vi "SetScale.vi"(8 "error in (no error)":errorcluster, 9 "Gauss":T1(ring), 10 "Arduino Resource In":T2={"VISA resource"="", "Board Type"=enum."Uno", "Connection Type"=enum."USB / Serial", "Bytes Per Packet (15)"=15}, 11 "HMC5883L in":refnum<class "HMC5883L.lvclass">) -> (0 "error out":errorcluster, 2 "Arduino Resource Out":T2={"VISA resource"="", "Board Type"=enum."Uno", "Connection Type"=enum."USB / Serial", "Bytes Per Packet (15)"=15}, 3 "HMC5883L out":refnum<class "HMC5883L.lvclass">)   [LabVIEW 2012, in "HMC5883L.lvclass"]
uses:
  HMC5883L.lvclass
  <vilib>/LabVIEW Interface for Arduino/LabVIEW Interface for Arduino.lvlib
  <vilib>/LabVIEW Interface for Arduino/Type Defs/Board Type.ctl
  <vilib>/LabVIEW Interface for Arduino/Type Defs/Arduino Resource.ctl
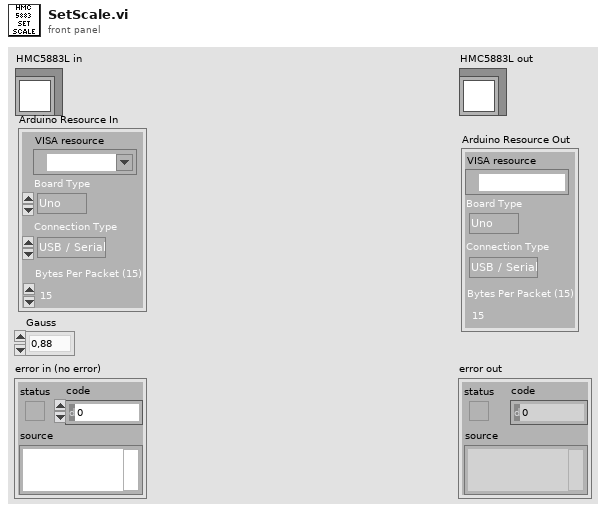
[diagram p1: front panel]
types:
  T1 = enum8{"0,88", "1,30", "1,90", "2,50", "4,00", "4,70", "5,60", "8,10"}
  T2 = typedef "LabVIEW Interface for Arduino.lvlib/Arduino Resource.ctl" = cluster{"VISA resource":refnum<visa-resource-name>, "Board Type":T3, "Connection Type":enum8{"USB / Serial"}, "Bytes Per Packet (15)":u8}
  T3 = typedef "LabVIEW Interface for Arduino.lvlib/Board Type.ctl" = enum16{"Uno", "Dimuelanove w/Atmega 328", "Mega 2560"}
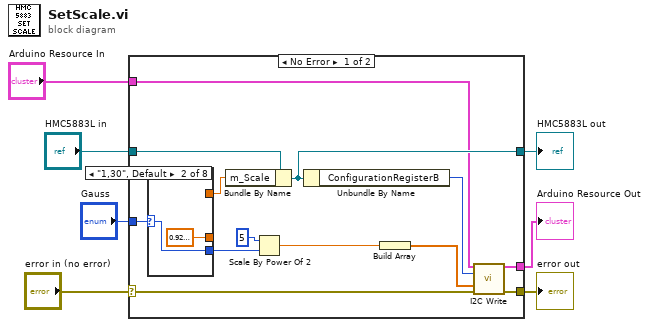
[diagram p0: block diagram]
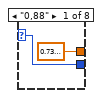
[diagram p2: hidden frame]
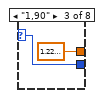
[diagram p3: hidden frame]
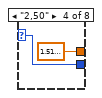
[diagram p4: hidden frame]
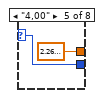
[diagram p5: hidden frame]
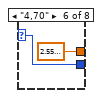
[diagram p6: hidden frame]
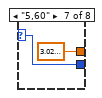
[diagram p7: hidden frame]
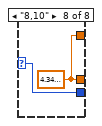
[diagram p8: hidden frame]
diagram:
  n1 = case shown="No Error" "error in (no error)" {
    selector: "error in (no error)" -> [w14 w39]
    tunnel: [w13 w39] -> w6
    tunnel: [w18 w38] -> w4
    tunnel: "HMC5883L in" -> [w20 w38]
    tunnel: "Arduino Resource In" -> [w16 w37]
    tunnel: [w15 w37] -> w2
    tunnel: "Gauss" -> [w10 _]
    frame No Error {
      n2 = case shown="\"1,30\", Default" w10 {
        selector: w10 -> [w21 w23 w25 w27 w29 w31 w33 w36]
        tunnel: [w21 w23 w25 w27 w29 w31 w33 w36] -> w9
        tunnel: [sgl 0.73 sgl 0.92 sgl 1.22 sgl 1.52 sgl 2.27 sgl 2.56 sgl 3.03 w35] -> _
        tunnel: [_ _ _ _ _ _ _ w35] -> w8
        frame "0,88" {
        }
        frame "1,30", Default {
        }
        frame "1,90" {
        }
        frame "2,50" {
        }
        frame "4,00" {
        }
        frame "4,70" {
        }
        frame "5,60" {
        }
        frame "8,10" {
          w35 = sgl 4.35
        }
      }
      n3 = Bundle By Name(cluster=w20, "m_Scale"=w8) -> (w18:refnum<class "HMC5883L.lvclass">)
      n4 = Scale By Power Of 2(n=i16 5, x=w9) -> (x*2^n=w12:dbl)
      n5 = Unbundle By Name(w18) -> ("ConfigurationRegisterB"=w17:u8)
      n6 = Build Array(w12) -> (w11:dbl[])
      n7 = call <vilib>:"I2C Write.vi"("Arduino Resource"=w16, "Address (0)"=w17, "I2C Data Bytes"=w11, "error in"=w14) -> ("Arduino Resource"=w15:T2, "error out"=w13:errorcluster)  [unwired: 10 in]
    }
    frame Error {
    }
  }
  "error out" <- w6
  "HMC5883L out" <- w4
  "Arduino Resource Out" <- w2
